vi "Clear.vi"(8 "error in (no error)":errorcluster, 11 "Slave Test Runner In":refnum<class "Slave Test Runner.lvclass">) -> (0 "error out":errorcluster, 3 "Slave Test Runner Out":refnum<class "Slave Test Runner.lvclass">)   [LabVIEW 2020, in "Slave Test Runner.lvclass"]
uses:
  Slave Test Runner.lvclass
  Application Framework/Process Classes/Process/Process.lvclass
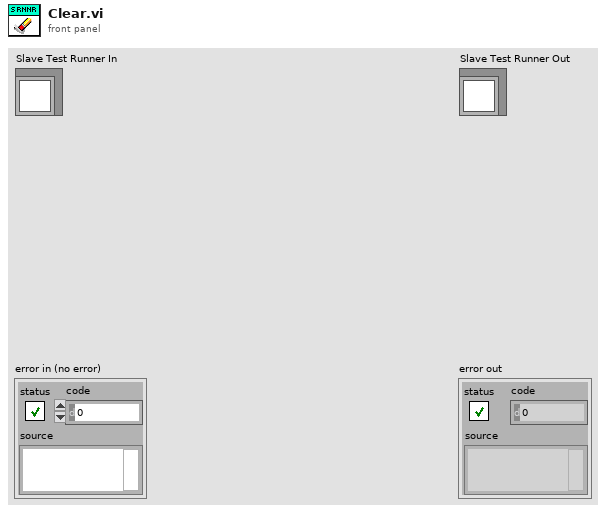
[diagram p1: front panel]
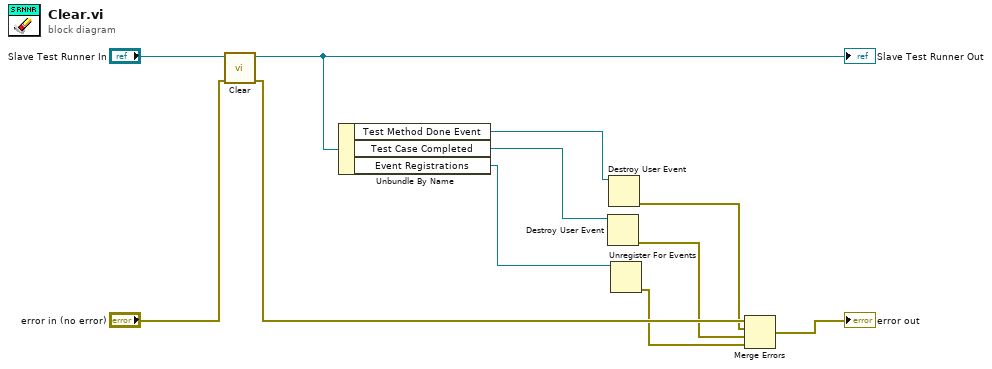
[diagram p0: block diagram]
diagram:
  n1 = call-parent "Clear.vi"("error in (no error)"="error in (no error)", "Process In"="Slave Test Runner In") -> ("error out"=w7:errorcluster, "Process Out"=w9:refnum<class "Slave Test Runner.lvclass">)  [unwired: 8 in]
  "Slave Test Runner Out" <- w9
  n2 = Unbundle By Name(w9) -> ("Test Method Done Event"=w4:refnum<user-event>, "Test Case Completed"=w6:refnum<user-event>, "Event Registrations"=w2:refnum<event-registration>)
  n3 = Destroy User Event(user event=w6) -> (error out=w5:errorcluster)  [unwired: 1 in]
  n4 = Destroy User Event(user event=w4) -> (error out=w3:errorcluster)  [unwired: 1 in]
  n5 = Unregister For Events(event registration refnum=w2) -> (error out=w1:errorcluster)  [unwired: 1 in]
  n6 = Merge Errors(w7, w3, w5, w1) -> (→"error out":errorcluster)
